vi "SaveRawFile.vi"(0 "FW Force Down":T1, 1 "MasterPath":path=path "D:/Output", 2 "EN":bool, 5 "RW Force Down":T1, 7 "FW Force Up":T1, 9 "RW Force Up":T1, 11 "Test Name":string(combo)="DL", 12 "OPC_FixtureData":u16[](array[numeric]), 13 "OPC_Model Type":u16 format="%x") -> (4 "Folder path":path, 8 "File path":path[](array[path]), 15 "SaveOK":bool)   [LabVIEW 2017]
uses:
  <vilib>/Utility/file.llb/Write Delimited Spreadsheet (string).vi
panel:
  # "DX = 4458\nK3 = 4B33\n4U = 3455\nWS = 5753\nL5 = 4C53\nKB = 4B42"
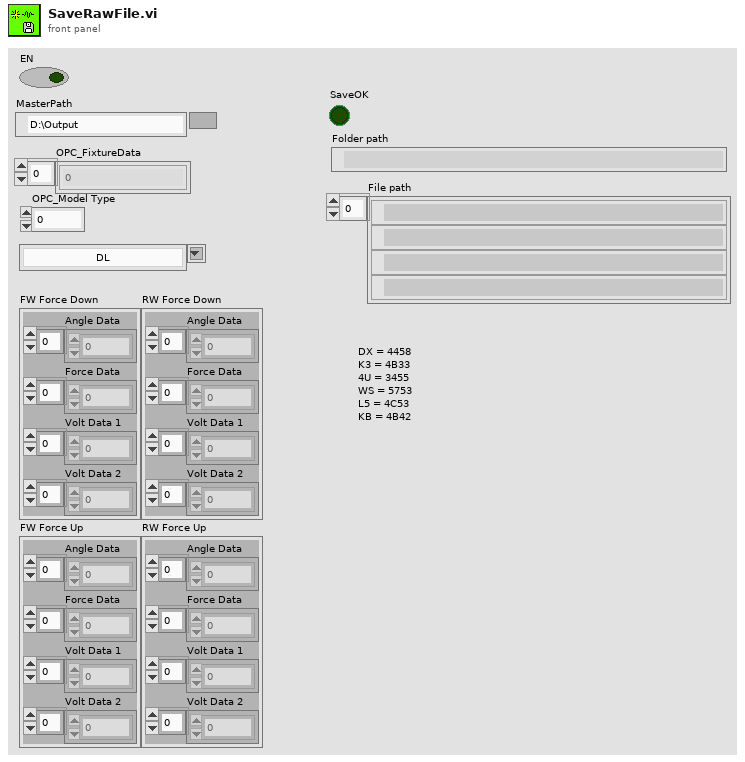
[diagram p1: front panel]
types:
  T1 = cluster{"Angle Data":dbl[], "Force Data":dbl[], "Volt Data 1":dbl[], "Volt Data 2":dbl[]}
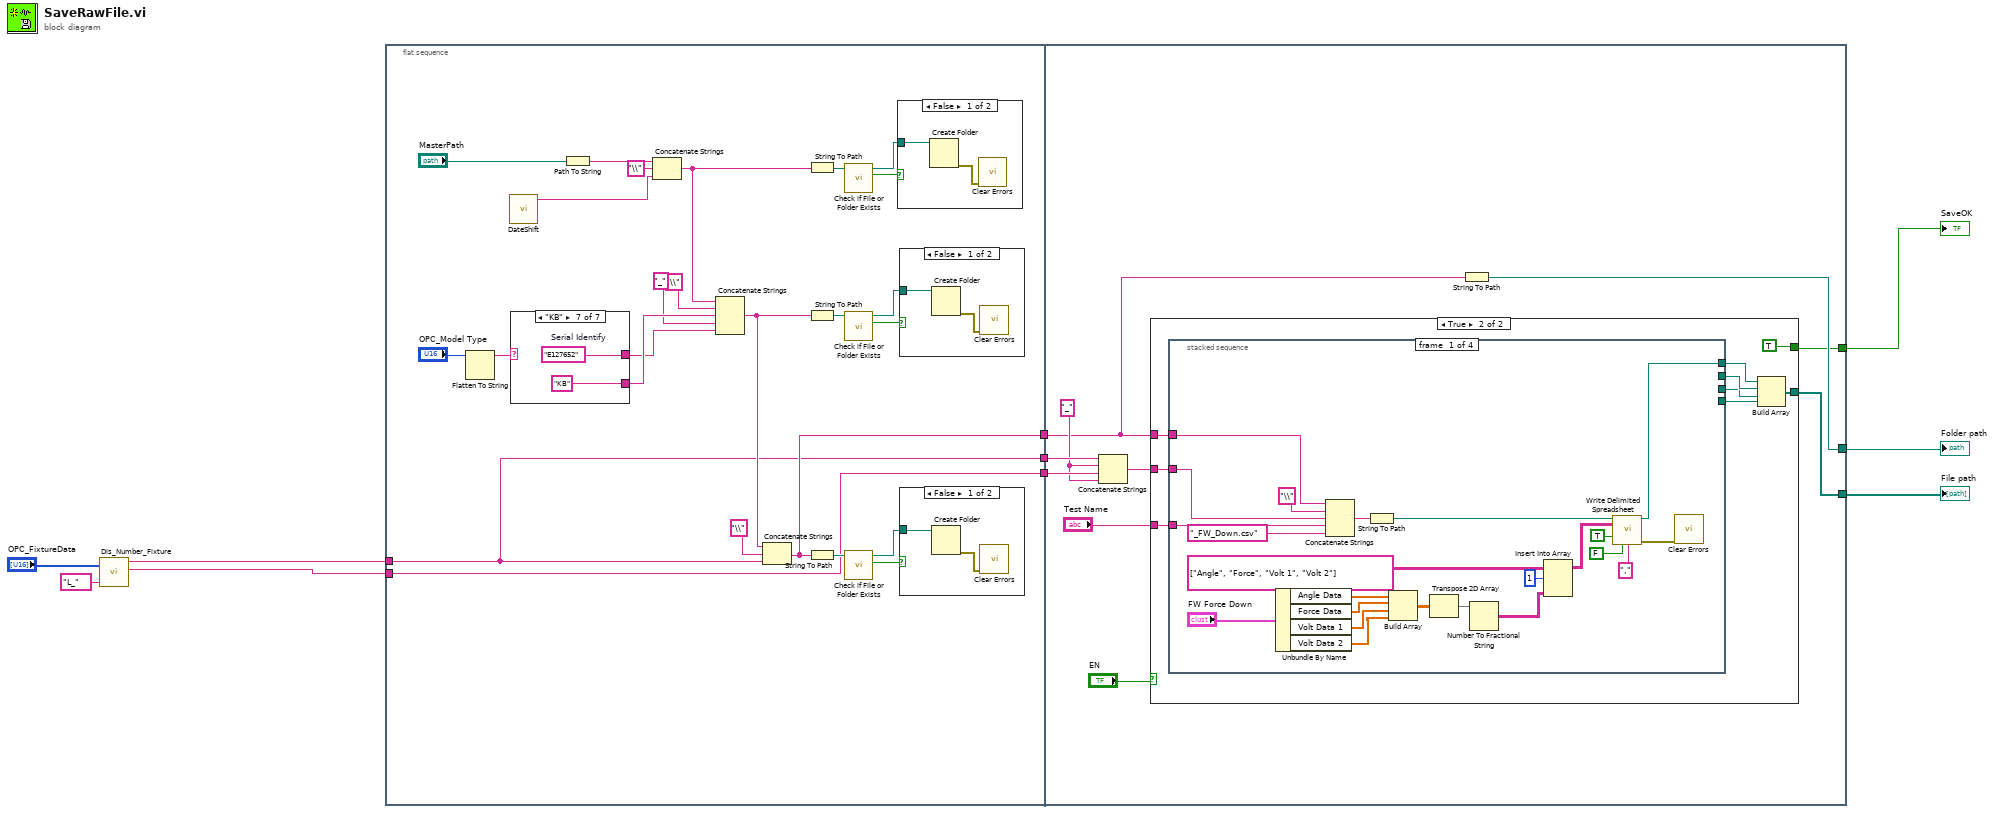
[diagram p0: block diagram]
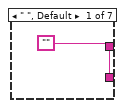
[diagram p4: hidden frame]
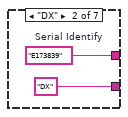
[diagram p5: hidden frame]
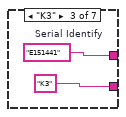
[diagram p6: hidden frame]
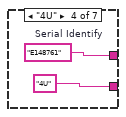
[diagram p7: hidden frame]
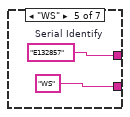
[diagram p8: hidden frame]
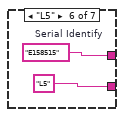
[diagram p9: hidden frame]
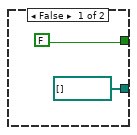
[diagram p11: hidden frame]
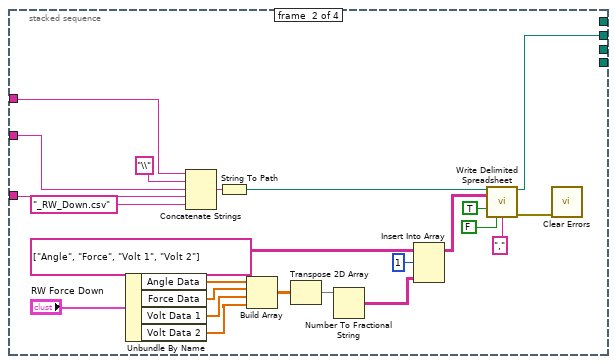
[diagram p12: hidden frame]
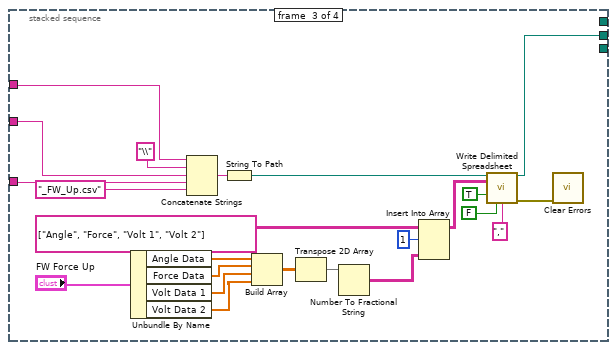
[diagram p13: hidden frame]
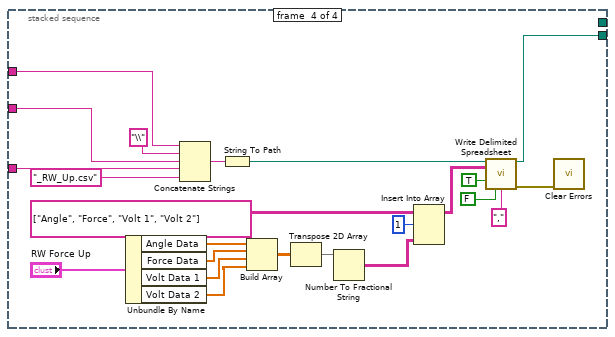
[diagram p14: hidden frame]
diagram:
  n1 = call "Dis_Number_Fixture.vi"("Lane Tyep"="L_", "Fixture_Data"="OPC_FixtureData") -> ("Lane Number"=w7:string, "Product Number"=w6:string)  [unwired: 5 in, 3 out]
  n2 = flat-sequence {
    tunnel: [w30] -> w3
    tunnel: [w12] -> w2
    tunnel: [w13] -> w1
    tunnel: w7 -> [w13]
    tunnel: w6 -> [w12]
    tunnel: w3 -> [w59]
    tunnel: w2 -> [w63]
    tunnel: w1 -> [w61]
    tunnel: [w57] -> w4
    tunnel: [w58] -> w10
    tunnel: [w55] -> w5
    frame #0 {
      n3 = Flatten To String(anything="OPC_Model Type") -> (data string=w28:string)  [unwired: 3 in, 2 out]
      n4 = call "DateShift.vi"() -> ("DateShift"=w11:string)  [unwired: 3 in, 2 out]
      n5 = case shown="\"KB\"" w28 {
        tunnel: [w40 w42 w44 w46 w48 w50 w52] -> w26
        tunnel: [w40 "DX" "K3" "4U" "WS" "L5" "KB"] -> w27
        frame " ", Default {
          w40 = ""
        }
        frame "DX" {
          w42 = "E173839"  # Serial Identify
        }
        frame "K3" {
          w44 = "E151441"  # Serial Identify
        }
        frame "4U" {
          w46 = "E148761"  # Serial Identify
        }
        frame "WS" {
          w48 = "E132857"  # Serial Identify
        }
        frame "L5" {
          w50 = "E158515"  # Serial Identify
        }
        frame "KB" {
          w52 = "E127652"  # Serial Identify
        }
      }
      n6 = Path To String(path="MasterPath") -> (string=w17:string)
      n7 = Concatenate Strings(w17, "\\" ("string"), w11) -> (w14:string)
      n8 = Concatenate Strings(w14, "\\" ("string"), w27, "_" ("string"), w26) -> (w31:string)
      n9 = Concatenate Strings(w31, "\\" ("string"), w12) -> (w30:string)
      n10 = String To Path(string=w14) -> (path=w19:path)
      n11 = String To Path(string=w31) -> (path=w24:path)
      n12 = String To Path(string=w30) -> (path=w34:path)
      n13 = call <vilib>:"Check if File or Folder Exists.vi"("path"=w19) -> ("file or folder exists?"=w20:bool, "dup path"=w21:path)  [unwired: 8 in, 1 out]
      n14 = call <vilib>:"Check if File or Folder Exists.vi"("path"=w24) -> ("file or folder exists?"=w23:bool, "dup path"=w22:path)  [unwired: 8 in, 1 out]
      n15 = call <vilib>:"Check if File or Folder Exists.vi"("path"=w34) -> ("file or folder exists?"=w33:bool, "dup path"=w32:path)  [unwired: 8 in, 1 out]
      n16 = case shown="False" w20 {
        tunnel: w21 -> [w37 _]
        frame False {
          n17 = Create Folder(path (use dialog)=w37) -> (error out=w36:errorcluster)  [unwired: 2 in, 2 out]
          n18 = call <vilib>:"Clear Errors.vi"("error in (no error)"=w36) -> ()  [unwired: 5 in, 2 out]
        }
        frame True {
        }
      }
      n19 = case shown="False" w23 {
        tunnel: w22 -> [w39 _]
        frame False {
          n20 = Create Folder(path (use dialog)=w39) -> (error out=w38:errorcluster)  [unwired: 2 in, 2 out]
          n21 = call <vilib>:"Clear Errors.vi"("error in (no error)"=w38) -> ()  [unwired: 5 in, 2 out]
        }
        frame True {
        }
      }
      n22 = case shown="False" w33 {
        tunnel: w32 -> [w54 _]
        frame False {
          n23 = Create Folder(path (use dialog)=w54) -> (error out=w53:errorcluster)  [unwired: 2 in, 2 out]
          n24 = call <vilib>:"Clear Errors.vi"("error in (no error)"=w53) -> ()  [unwired: 5 in, 2 out]
        }
        frame True {
        }
      }
    }
    frame #1 {
      w60 = "_" ("string")
      n25 = Concatenate Strings(w63, w60, w61, w60) -> (w62:string)
      n26 = case shown="True" "EN" {
        tunnel: "Test Name" -> [_ w75]
        tunnel: w62 -> [_ w74]
        tunnel: w59 -> [_ w73]
        tunnel: [path[] [] w71] -> w57
        tunnel: [FALSE TRUE] -> w55
        frame False {
        }
        frame True {
          n27 = stacked-sequence {
            tunnel: w75 -> [w93 w103 w123 w150]
            tunnel: w74 -> [w79 w102 w124 w148]
            tunnel: w73 -> [w77 w101 w125 w147]
            tunnel: [w76 _ _ _] -> w72
            tunnel: [_ w99 _ _] -> w70
            tunnel: [_ _ w122 _] -> w69
            tunnel: [_ _ _ w145] -> w68
            frame #0 {
              n28 = Unbundle By Name("FW Force Down") -> ("Angle Data"=w84:dbl[], "Force Data"=w85:dbl[], "Volt Data 1"=w86:dbl[], "Volt Data 2"=w87:dbl[])
              n29 = Concatenate Strings(w77, "\\" ("string"), w79, w93, "_FW_Down.csv" ("string")) -> (w95:string)
              n30 = String To Path(string=w95) -> (path=w94:path)
              n31 = Build Array(w84, w85, w86, w87) -> (w88:dbl[][])
              n32 = Transpose 2D Array(2D array=w88) -> (transposed array=w89:dbl[][])
              n33 = Number To Fractional String(number=w89) -> (F-format string=w90:string[][])  [unwired: 3 in]
              n34 = Insert Into Array(array=string[][] [["Angle", "Force", "Volt 1", "Volt 2"]], index (row)=1, new element=w90) -> (w81:string[][])  [unwired: 1 in]
              n35 = call-poly <vilib>:"Write Delimited Spreadsheet.vi"("file path (dialog if empty)"=w94, "2D data"=w81, "append to file? (new file:F)"=TRUE, "transpose? (no:F)"=FALSE, "delimiter (\\t)"="," ("delimiter (\\t)")) -> ("new file path (Not A Path if cancelled)"=w76:path, "error out"=w80:errorcluster)  [unwired: 9 in]
              n36 = call <vilib>:"Clear Errors.vi"("error in (no error)"=w80) -> ()  [unwired: 5 in, 2 out]
            }
            frame #1 {
              n37 = Unbundle By Name("RW Force Down") -> ("Angle Data"=w110:dbl[], "Force Data"=w111:dbl[], "Volt Data 1"=w112:dbl[], "Volt Data 2"=w113:dbl[])
              n38 = Concatenate Strings(w101, "\\" ("string"), w102, w103, "_RW_Down.csv" ("string")) -> (w100:string)
              n39 = String To Path(string=w100) -> (path=w118:path)
              n40 = Build Array(w110, w111, w112, w113) -> (w114:dbl[][])
              n41 = Transpose 2D Array(2D array=w114) -> (transposed array=w115:dbl[][])
              n42 = Number To Fractional String(number=w115) -> (F-format string=w116:string[][])  [unwired: 3 in]
              n43 = Insert Into Array(array=string[][] [["Angle", "Force", "Volt 1", "Volt 2"]], index (row)=1, new element=w116) -> (w107:string[][])  [unwired: 1 in]
              n44 = call-poly <vilib>:"Write Delimited Spreadsheet.vi"("file path (dialog if empty)"=w118, "2D data"=w107, "append to file? (new file:F)"=TRUE, "transpose? (no:F)"=FALSE, "delimiter (\\t)"="," ("delimiter (\\t)")) -> ("new file path (Not A Path if cancelled)"=w99:path, "error out"=w106:errorcluster)  [unwired: 9 in]
              n45 = call <vilib>:"Clear Errors.vi"("error in (no error)"=w106) -> ()  [unwired: 5 in, 2 out]
            }
            frame #2 {
              n46 = Unbundle By Name("FW Force Up") -> ("Angle Data"=w134:dbl[], "Force Data"=w135:dbl[], "Volt Data 1"=w136:dbl[], "Volt Data 2"=w137:dbl[])
              n47 = Concatenate Strings(w125, "\\" ("string"), w124, w123, "_FW_Up.csv" ("string")) -> (w127:string)
              n48 = String To Path(string=w127) -> (path=w141:path)
              n49 = Build Array(w134, w135, w136, w137) -> (w138:dbl[][])
              n50 = Transpose 2D Array(2D array=w138) -> (transposed array=w139:dbl[][])
              n51 = Number To Fractional String(number=w139) -> (F-format string=w140:string[][])  [unwired: 3 in]
              n52 = Insert Into Array(array=string[][] [["Angle", "Force", "Volt 1", "Volt 2"]], index (row)=1, new element=w140) -> (w131:string[][])  [unwired: 1 in]
              n53 = call-poly <vilib>:"Write Delimited Spreadsheet.vi"("file path (dialog if empty)"=w141, "2D data"=w131, "append to file? (new file:F)"=TRUE, "transpose? (no:F)"=FALSE, "delimiter (\\t)"="," ("delimiter (\\t)")) -> ("new file path (Not A Path if cancelled)"=w122:path, "error out"=w129:errorcluster)  [unwired: 9 in]
              n54 = call <vilib>:"Clear Errors.vi"("error in (no error)"=w129) -> ()  [unwired: 5 in, 2 out]
            }
            frame #3 {
              n55 = Unbundle By Name("RW Force Up") -> ("Angle Data"=w157:dbl[], "Force Data"=w158:dbl[], "Volt Data 1"=w159:dbl[], "Volt Data 2"=w160:dbl[])
              n56 = Concatenate Strings(w147, "\\" ("string"), w148, w150, "_RW_Up.csv" ("string")) -> (w149:string)
              n57 = String To Path(string=w149) -> (path=w164:path)
              n58 = Build Array(w157, w158, w159, w160) -> (w161:dbl[][])
              n59 = Transpose 2D Array(2D array=w161) -> (transposed array=w162:dbl[][])
              n60 = Number To Fractional String(number=w162) -> (F-format string=w163:string[][])  [unwired: 3 in]
              n61 = Insert Into Array(array=string[][] [["Angle", "Force", "Volt 1", "Volt 2"]], index (row)=1, new element=w163) -> (w153:string[][])  [unwired: 1 in]
              n62 = call-poly <vilib>:"Write Delimited Spreadsheet.vi"("file path (dialog if empty)"=w164, "2D data"=w153, "append to file? (new file:F)"=TRUE, "transpose? (no:F)"=FALSE, "delimiter (\\t)"="," ("delimiter (\\t)")) -> ("new file path (Not A Path if cancelled)"=w145:path, "error out"=w146:errorcluster)  [unwired: 9 in]
              n63 = call <vilib>:"Clear Errors.vi"("error in (no error)"=w146) -> ()  [unwired: 5 in, 2 out]
            }
          }
          n64 = Build Array(w72, w70, w69, w68) -> (w71:path[])
        }
      }
      n65 = String To Path(string=w59) -> (path=w58:path)
    }
  }
  "Folder path" <- w10
  "SaveOK" <- w5
  "File path" <- w4
